vi "Update Series DVR U16.vi"(8 "error in (no error)":errorcluster, 9 "Image #":u32, 10 "image ref array":refnum<data-value>[](array[refnum]), 11 "Series Graph in":refnum<class "Series Graph.lvclass">) -> (0 "error out":errorcluster, 3 "Series Graph out":refnum<class "Series Graph.lvclass">)   [LabVIEW 2023, in "Series Graph.lvclass"]
uses:
  Series Graph.lvclass
  Series Graph.lvclass/Series Graph.ctl
  Detail Graph/Detail Graph.lvclass
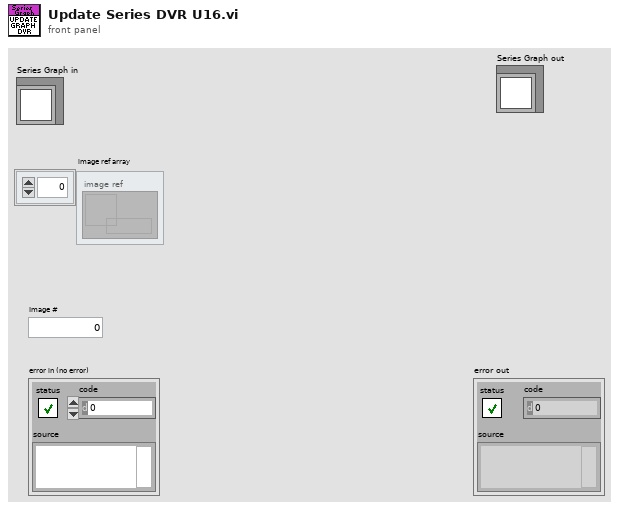
[diagram p1: front panel]
types:
  T1 = typedef "LVPointDoubleTypeDef.ctl" = cluster{"X":dbl, "Y":dbl}
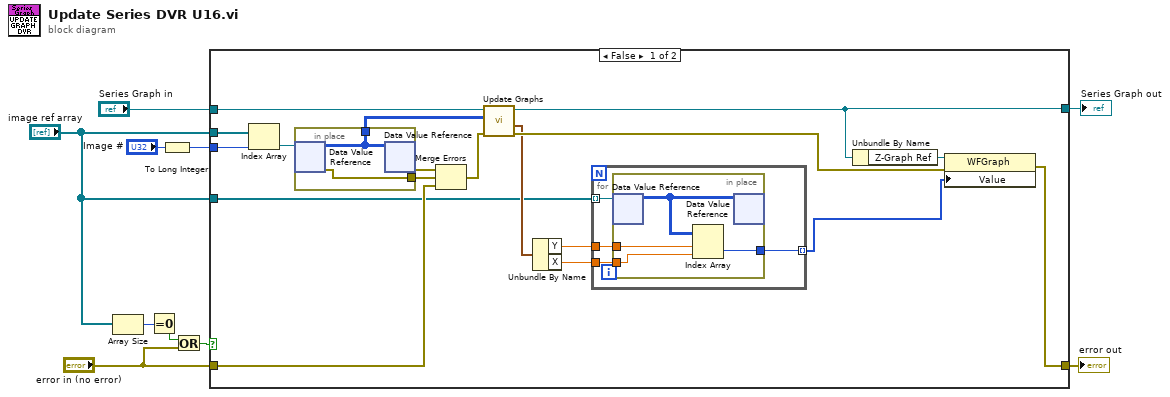
[diagram p0: block diagram]
diagram:
  n1 = Array Size(array="image ref array") -> (size(s)=w2:i32)
  n2 = Equal To 0?(x=w2) -> (x = 0?=w8:bool)
  n3 = To Long Integer(number="Image #") -> (32bit integer=w3:i32)
  n4 = Or(x=w8, y="error in (no error)") -> (x .or. y?=w9:bool)
  n5 = case shown="False" w9 {
    tunnel: [w27 w40] -> w10
    tunnel: [w16 w39] -> w4
    tunnel: w3 -> [w24 _]
    tunnel: "error in (no error)" -> [w18 w40]
    tunnel: "Series Graph in" -> [w25 w39]
    tunnel: "image ref array" -> [w23 _]
    tunnel: "image ref array" -> [w14 _]
    frame False {
      n6 = Index Array(array=w23, index=w24) -> (element=w22:refnum<data-value>)
      n7 = in-place {
        in-place-border: [w38] -> w21
        in-place-border: [w37] -> w17
        n8 = in-place-dvr #1(w22) -> (w38:u16[][], w37:errorcluster)
        n9 = in-place-dvr #1(w38) -> (w20:errorcluster)  [unwired: 1 out]
      }
      n10 = Merge Errors(w20, w17, w18) -> (w19:errorcluster)
      n11 = call "Update Graphs.vi"("error in (no error)"=w19, "image"=w21, "Detail Graph in"=w25) -> ("error out"=w28:errorcluster, "Cursor.Cursor Position"=w26:T1, "Detail Graph out"=w16:refnum<class "Series Graph.lvclass">)  [unwired: 6 in]
      n12 = Unbundle By Name(w26) -> ("Y"=w13:dbl, "X"=w12:dbl)
      n13 = for {
        tunnel: w14 -> [w32] mode=indexing
        tunnel: w13 -> [w31]
        tunnel: w12 -> [w30]
        tunnel: [w29] -> w11 mode=indexing
        n14 = in-place {
          in-place-border: w31 -> [w36]
          in-place-border: w30 -> [w35]
          in-place-border: [w34] -> w29
          n15 = in-place-dvr #2(w32) -> (w33:u16[][])  [unwired: 1 out]
          n16 = Index Array(array=w33, index (row)=w36, index (col)=w35) -> (element=w34:u16)
          n17 = in-place-dvr #2(w33) -> ()  [unwired: 2 out]
        }
      }
      n18 = Unbundle By Name(w16) -> ("Z-Graph Ref"=w15:refnum<vi>)
      n19 = property class="WFGraph"(reference=w15, error in=w28, "Value"=w11) -> (error out=w27:errorcluster)  [unwired: 1 out]
    }
    frame True {
    }
  }
  "error out" <- w10
  "Series Graph out" <- w4
